vi "Set main screen Objective control index.vi"(8 "error in (no error)":errorcluster, 11 "Objective control index":i32) -> (0 "error out":errorcluster, 3 "Changed?":bool)   [LabVIEW 2020]
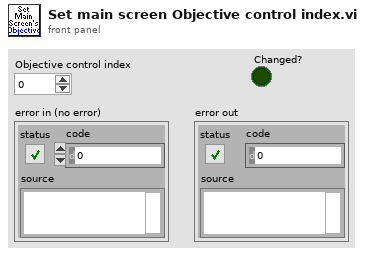
[diagram p1: front panel]
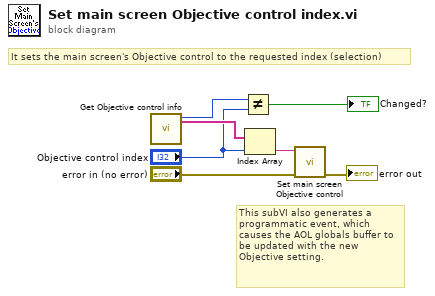
[diagram p0: block diagram]
diagram:
  # "This subVI also generates a programmatic event, which causes the AOL globals buffer to be updated with the new Objective setting."
  # "It sets the main screen's Objective control to the requested index (selection)"
  n1 = call "Get Objective control info.vi"() -> ("Selection index"=w2:i32, "Objective values/strings"=w5:string[])  [unwired: 7 in, 3 out]
  n2 = Not Equal?(x=w2, y="Objective control index") -> (x != y?=→"Changed?":bool)
  n3 = Index Array(array=w5, index="Objective control index") -> (element=w4:string)
  n4 = call "Set main screen Objective control.vi"("error in (no error)"="error in (no error)", "Objective value (Signaling)"=w4) -> ("error out"=→"error out":errorcluster)  [unwired: 9 in]
